vi "Get Menu Commands.vi"(8 "error in (no error)":errorcluster, 9 "Active Build Configuration":string, 10 "Selected Items":string[][](array[string]), 11 "ZIP Item in":refnum<class "ZIP Item.lvclass">) -> (0 "error out":errorcluster, 2 "Menu":string[](array[string]))   [LabVIEW 2019, in "ZIP.lvlib" / "ZIP Item.lvclass"]
uses:
  ZIP Item.lvclass
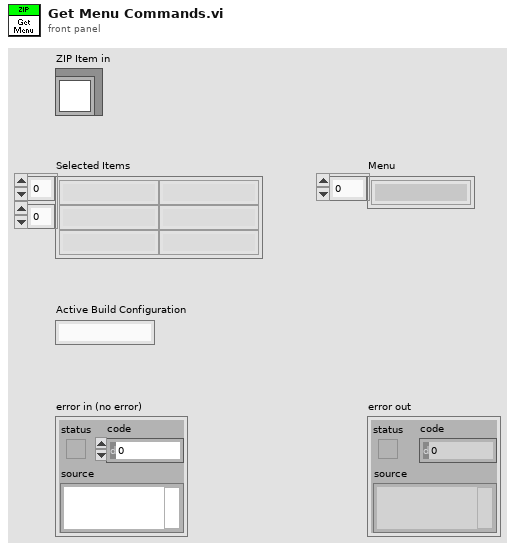
[diagram p1: front panel]
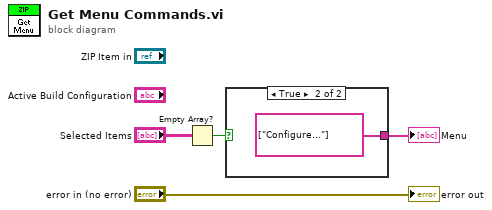
[diagram p0: block diagram]
diagram:
  n1 = Empty Array?(array="Selected Items") -> (empty?=w2:bool)
  n2 = case shown="True" w2 {
    tunnel: [_ string[] ["Configure..."] ("Menu")] -> w3
    frame False {
    }
    frame True {
    }
  }
  "Menu" <- w3
  "error out" <- "error in (no error)"
